vi "filter_color.vi"(9 "exclude color":u32(colorbox), 10 "input":T1[](array[typedef])) -> (2 "output":T1[](array[typedef]))   [LabVIEW 2023]
uses:
  pixel.ctl
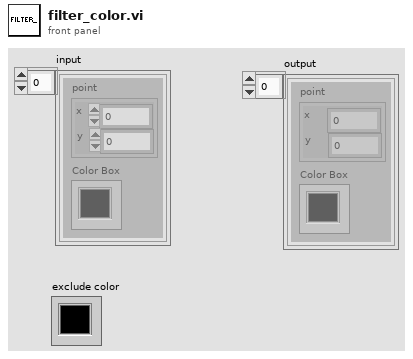
[diagram p1: front panel]
types:
  T1 = typedef "pixel.ctl" = cluster{"point":cluster{"x":i16, "y":i16}, "Color Box":u32}
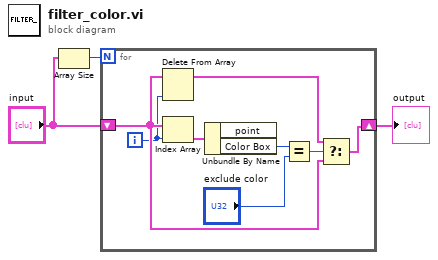
[diagram p0: block diagram]
diagram:
  n1 = Array Size(array="input") -> (size(s)=w1:i32)
  n2 = for {
    N: w1 -> [_]
    shift-right: [w4] -> w3
    shift-left: "input" -> [w7]
    i -> [w6]
    n3 = Delete From Array(array=w7, index=w6) -> (array with subset deleted=w5:T1[])  [unwired: 1 in, 1 out]
    n4 = Index Array(array=w7, index=w6) -> (element=w11:T1)
    n5 = Unbundle By Name(w11) -> ("Color Box"=w9:u32)  [unwired: 1 out]
    n6 = Equal?(x=w9, y="exclude color") -> (x = y?=w8:bool)
    n7 = Select(t=w5, s=w8, f=w7) -> (s? t:f=w4:T1[])
  }
  "output" <- w3
